vi "Rinocloud_lab_simulator.vi"() -> ()   [LabVIEW 2011, in "Rinocloud Library.lvlib"]
uses:
  Rinocloud Library.lvlib
  <vilib>/Utility/miscctls.llb/LVDateTimeRec.ctl
  Rinocloud_global_variable.vi
panel:
  in  "Active item:":string
  in  "image":bool
  out "Data saved":bool
  in  "extra information field 2":T1={"Attribute"="Sample ID", "Value"="A2008", "Data type"=enum."String"}
  in  "extra information field 3":T1={"Attribute"="Units", "Value"="nm,cps", "Data type"=enum."1D array of strings"}
  in  "notes":string="Rino client testing"
  in  "tags":string="1D data, testing"
  in  "name":string="Measurements"
  in  "extra information field":T1={"Attribute"="Labels", "Value"="Timestamp,Amplitude", "Data type"=enum."1D array of strings"}
  out "data JSON string":string="[[], []]"
  in  "Run":bool
  in  "Save":bool
  in  "X axis type:":u16(ring) items=["numerical"]
  out "headers":string
  out "body":string
  out "XY Graph":cluster{"x axis":dbl[], "x axis":dbl[]}[](graph)
  out "output array":cluster{"x axis":dbl[], "2D data":dbl[]}[](array[cluster])
  out "x axis":dbl[](array[numeric])
  out "1D data":dbl[](array[numeric])
  out "Array":dbl[](array[numeric])
  out "z axis":dbl[](array[numeric])
  out "2D data":dbl[][](array[numeric])
  out "x timestamps":string[](array[string])
  out "x native timestamp":timestamp[](array[timestamp])
  in  "stop":bool
  in  "Data type:":u16(ring) items=["1D array", "2D array"]
  # ":"
  # "{\"Attribute\" : \"Value\"}"
  # ":"
  # "{\"Attribute\" : \"Value\"}"
  # ":"
  # "{\"Attribute\" : \"Value\"}"
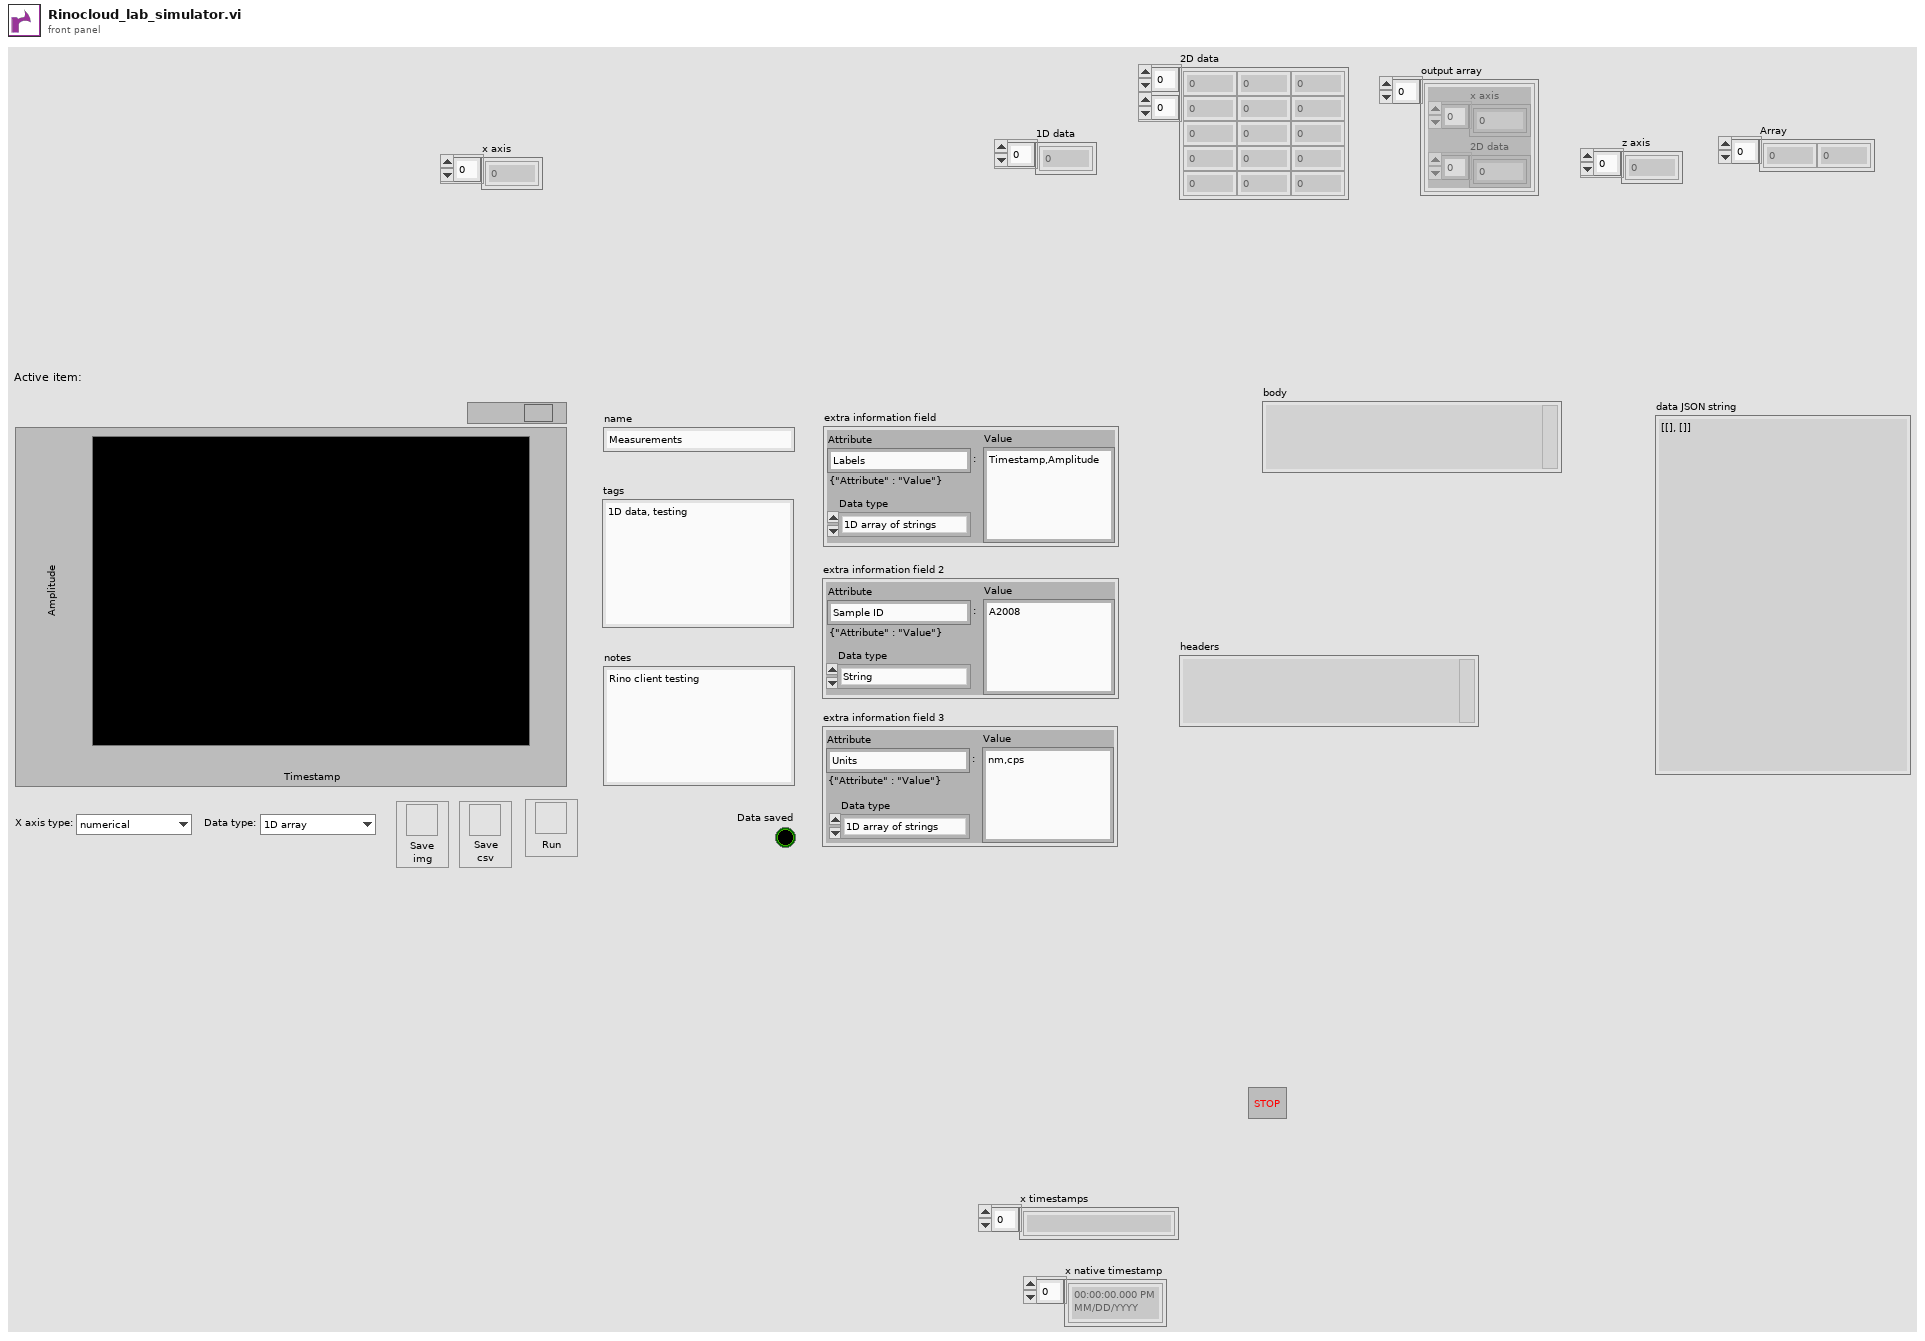
[diagram p1: front panel]
types:
  T1 = cluster{"Attribute":string, "Value":string, "Data type":enum16{"Numeric", "String", "1D array of strings", "1D array of doubles", "Data JSON string", "<null>"}}
  T2 = typedef "LVDateTimeRec.ctl" = cluster{"fractional second":dbl, "second":i32, "minute":i32, "hour":i32, "day of month":i32, "month":i32, "year":i32, "day of week":i32, "day of year":i32, "DST":i32}
  T3 = cluster{"Attribute":string, "Value":string, "Data type":enum16{"Numeric", "String", "1D array of strings", "1D array of doubles", "Data JSON string", "<null>"}}[]
  T4 = cluster{"headers":string, "body":string, "ID":string, "Saved":bool}
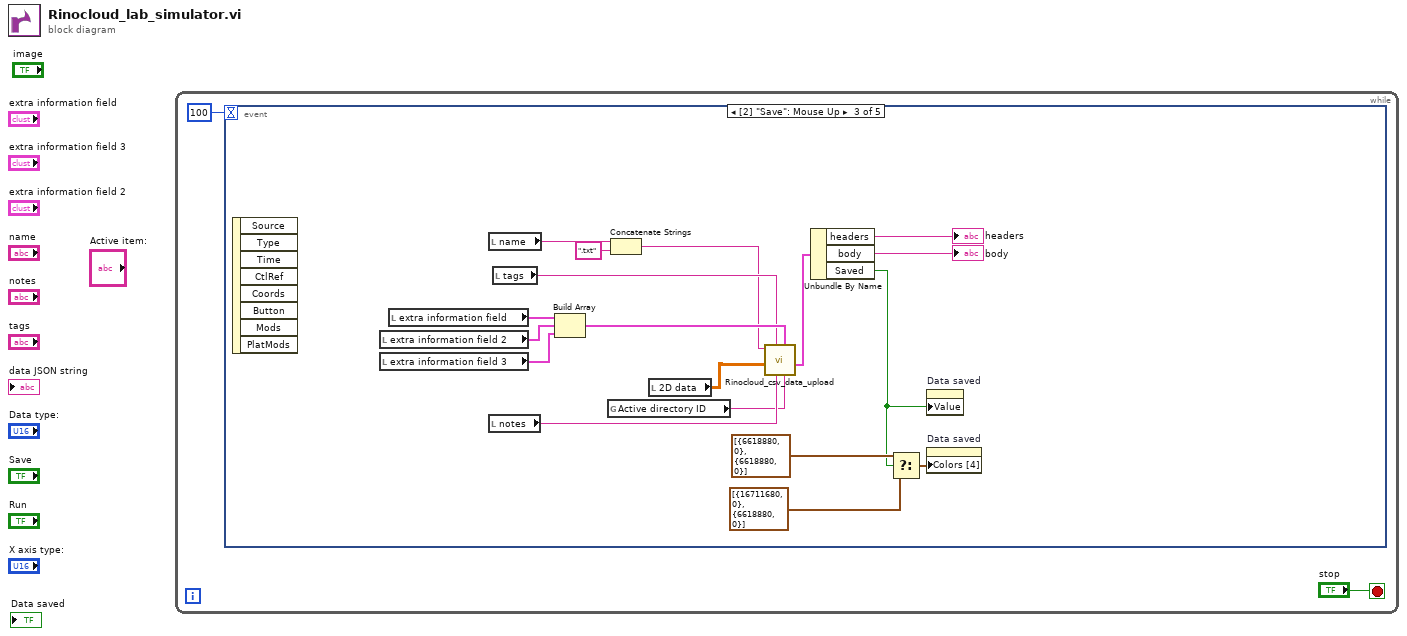
[diagram p0: block diagram]
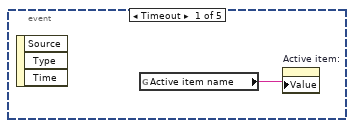
[diagram p2: hidden frame]
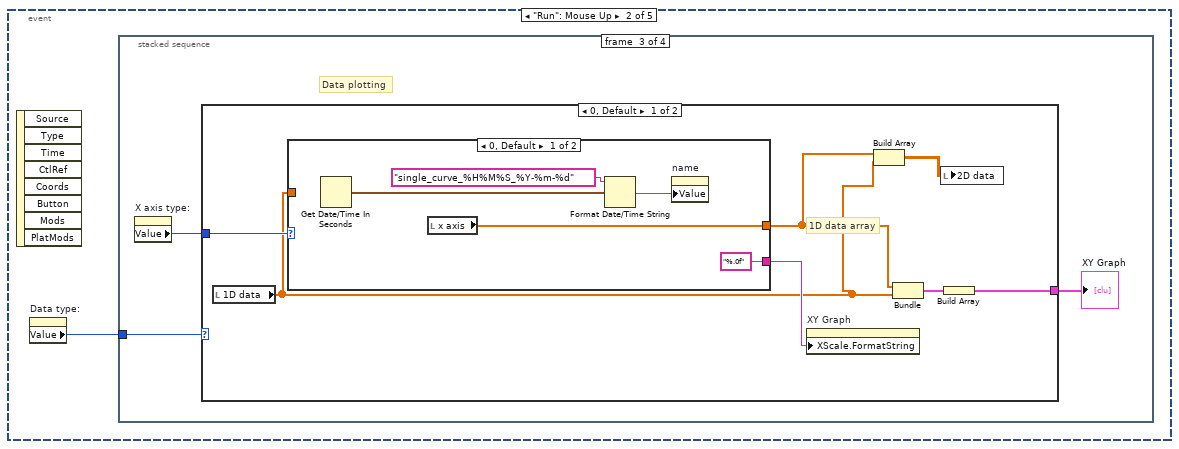
[diagram p3: hidden frame]
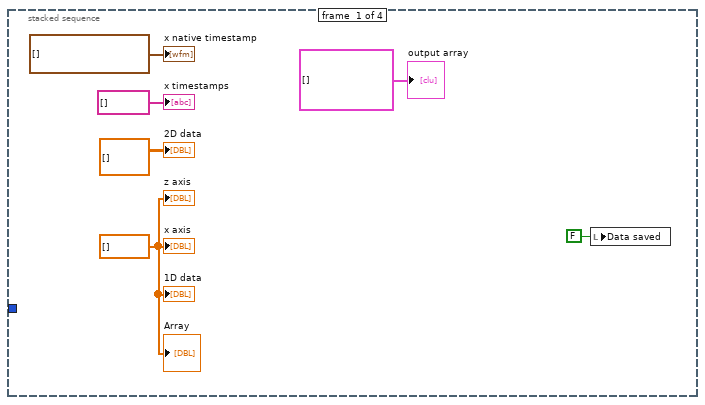
[diagram p4: hidden frame]
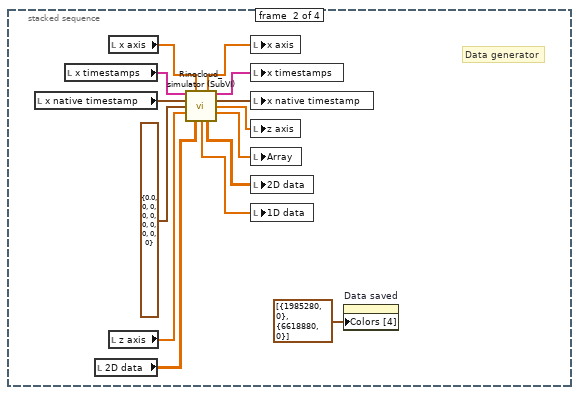
[diagram p5: hidden frame]
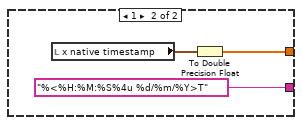
[diagram p6: hidden frame]
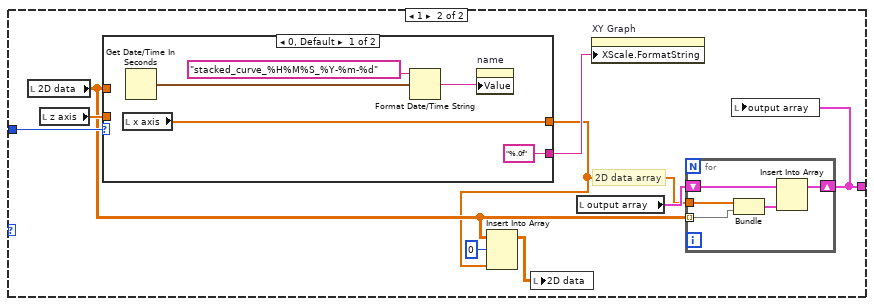
[diagram p7: hidden frame]
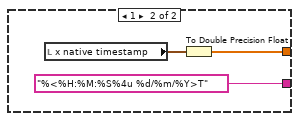
[diagram p8: hidden frame]
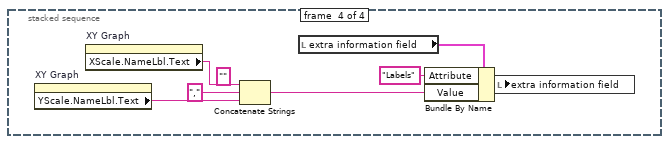
[diagram p9: hidden frame]
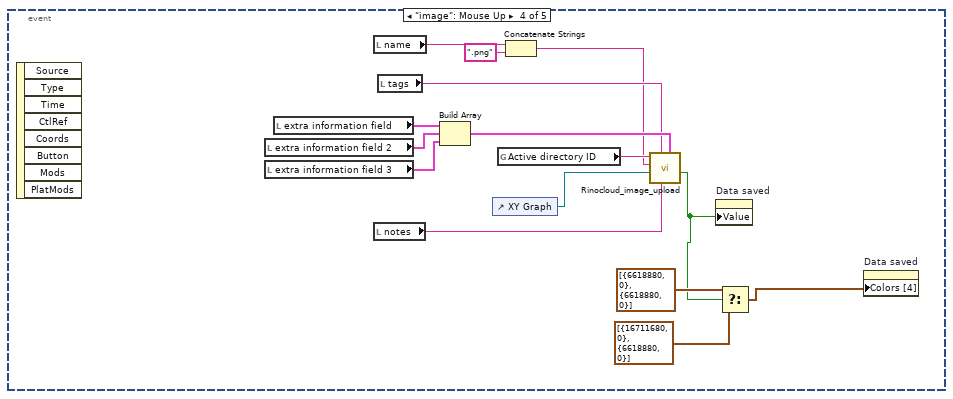
[diagram p10: hidden frame]
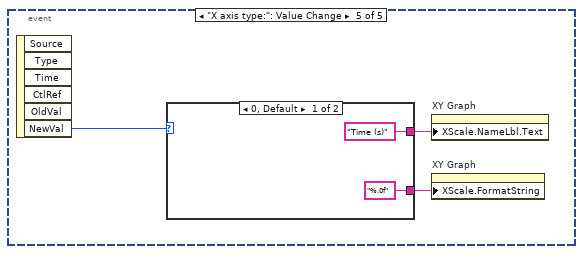
[diagram p11: hidden frame]
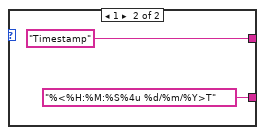
[diagram p12: hidden frame]
diagram:
  n1 = while {
    stop <- "stop" stop-if-true
    n2 = event shown="[2] \"Save\": Mouse Up" {
      selector: _ -> [_ _ _ _ _]
      dyn-events: _ -> [_ _ _ _ _]
      timeout: 100 -> [_ _ _ _ _]
      event Timeout {
        n3 = event-data() -> ()  [unwired: 1 in, 3 out]
        n4 = global read "Rinocloud_global_variable.vi" "Active item name"() -> (w3:string)
        n5 = property on="Active item:" class="Str"("Value"=w3) -> ()  [unwired: 2 in, 2 out]
      }
      event "Run": Mouse Up {
        n6 = event-data() -> ()  [unwired: 1 in, 8 out]
        n7 = property on="Data type:" class="Ring (strict)"() -> ("Value"=w4:u16)  [unwired: 2 in, 2 out]
        n8 = stacked-sequence {
          tunnel: w4 -> [_ _ w27 _]
          frame #0 {
            w9 = dbl[] []
            n9 = local write "Data saved"(FALSE ("Data saved")) -> ()
            "output array" <- cluster{"x axis":dbl[], "2D data":dbl[]}[] [] ("output array")
            "x axis" <- w9
            "1D data" <- w9
            "Array" <- w9
            "z axis" <- w9
            "2D data" <- dbl[][] []
            "x timestamps" <- string[] [] ("x timestamps")
            "x native timestamp" <- timestamp[] [] ("x native timestamp")
          }
          frame #1 {
            # "Data generator"
            n10 = local read "x native timestamp"() -> (w14:timestamp[])
            n11 = local read "x timestamps"() -> (w16:string[])
            n12 = local read "2D data"() -> (w23:dbl[][])
            n13 = local read "x axis"() -> (w24:dbl[])
            n14 = local read "z axis"() -> (w18:dbl[])
            n15 = call "Rinocloud_simulator (SubVI).vi"("x timestamps in"=w16, "x axis in"=w24, "x native timestamp in"=w14, "date time rec"=T2 {"fractional second"=0.0, "second"=0, "minute"=0, "hour"=0, "day of month"=0, "month"=0, "year"=0, "day of week"=0, "day of year"=0, "DST"=0}, "z axis in"=w18, "2D data in"=w23) -> ("x axis out"=w19:dbl[], "x timestamps out"=w15:string[], "x native timestamp out"=w13:timestamp[], "z axis out"=w17:dbl[], "Array 2"=w21:dbl[], "Array"=w20:dbl[], "2D data out"=w22:dbl[][])  [unwired: 3 in]
            n16 = local write "x axis"(w19) -> ()
            n17 = local write "x timestamps"(w15) -> ()
            n18 = local write "x native timestamp"(w13) -> ()
            n19 = local write "z axis"(w17) -> ()
            n20 = local write "Array"(w21) -> ()
            n21 = local write "2D data"(w22) -> ()
            n22 = local write "1D data"(w20) -> ()
            n23 = property on="Data saved" class="Bool (strict)"("Colors [4]"=cluster{u32, u32}[] [{1985280, 0}, {6618880, 0}]) -> ()  [unwired: 2 in, 2 out]
          }
          frame #2 {
            # "Data plotting"
            n24 = property on="X axis type:" class="Ring (strict)"() -> ("Value"=w25:u16)  [unwired: 2 in, 2 out]
            n25 = case shown="0, Default" w27 {
              tunnel: [w33 w50] -> w26
              tunnel: w25 -> [w32 w48]
              frame 0, Default {
                # "1D data array"
                n26 = local read "1D data"() -> (w29:dbl[])
                n27 = case shown="0, Default" w32 {
                  tunnel: [w38 w40] -> w30
                  tunnel: ["%.0f" ("X Scale.Format String") "%<%H:%M:%S%4u %d/%m/%Y>T" ("X Scale.Format String")] -> w31
                  tunnel: w29 -> [_ _]
                  frame 0, Default {
                    n28 = Get Date/Time In Seconds() -> (seconds since 1Jan1904=w37:timestamp)
                    n29 = local read "x axis"() -> (w38:dbl[])
                    n30 = Format Date/Time String(time format string (%c)="single_curve_%H%M%S_%Y-%m-%d", seconds (now)=w37) -> (date/time string=w36:string)  [unwired: 1 in]
                    n31 = property on="name" class="Str"("Value"=w36) -> ()  [unwired: 2 in, 2 out]
                  }
                  frame 1 {
                    n32 = local read "x native timestamp"() -> (w41:timestamp[])
                    n33 = To Double Precision Float(number=w41) -> (double precision float=w40:dbl[])
                  }
                }
                n34 = property on="XY Graph" class="XYGraph (strict)"("XScale.FormatString"=w31) -> ()  [unwired: 2 in, 2 out]
                n35 = Build Array(w30, w29) -> (w28:dbl[][])
                n36 = Bundle("x axis"=w30, "1D data"=w29) -> (w34:cluster{"x axis":dbl[], "1D data":dbl[]})  [unwired: 1 in]
                n37 = local write "2D data"(w28) -> ()
                n38 = Build Array(w34) -> (w33:cluster{"x axis":dbl[], "1D data":dbl[]}[])
              }
              frame 1 {
                # "2D data array"
                n39 = local read "2D data"() -> (w44:dbl[][])
                n40 = local read "z axis"() -> (w47:dbl[])
                n41 = case shown="0, Default" w48 {
                  tunnel: [w55 w57] -> w43
                  tunnel: ["%.0f" ("X Scale.Format String") "%<%H:%M:%S%4u %d/%m/%Y>T" ("X Scale.Format String")] -> w49
                  tunnel: w47 -> [_ _]
                  tunnel: w44 -> [_ _]
                  frame 0, Default {
                    n42 = local read "x axis"() -> (w55:dbl[])
                    n43 = Get Date/Time In Seconds() -> (seconds since 1Jan1904=w53:timestamp)
                    n44 = Format Date/Time String(time format string (%c)="stacked_curve_%H%M%S_%Y-%m-%d", seconds (now)=w53) -> (date/time string=w52:string)  [unwired: 1 in]
                    n45 = property on="name" class="Str"("Value"=w52) -> ()  [unwired: 2 in, 2 out]
                  }
                  frame 1 {
                    n46 = local read "x native timestamp"() -> (w58:timestamp[])
                    n47 = To Double Precision Float(number=w58) -> (double precision float=w57:dbl[])
                  }
                }
                n48 = Insert Into Array(array=w44, index (row)=0, new element=w43) -> (w46:dbl[][])  [unwired: 1 in]
                n49 = local write "2D data"(w46) -> ()
                n50 = local read "output array"() -> (w51:cluster{"x axis":dbl[], "2D data":dbl[]}[])
                n51 = property on="XY Graph" class="XYGraph (strict)"("XScale.FormatString"=w49) -> ()  [unwired: 2 in, 2 out]
                n52 = for {
                  tunnel: w44 -> [w63] mode=indexing
                  tunnel: w43 -> [w64]
                  shift-right: [w61] -> w50
                  shift-left: w51 -> [w60]
                  n53 = Bundle("x axis"=w64, "2D data"=w63) -> (w62:cluster{"x axis":dbl[], "2D data":dbl[]})  [unwired: 1 in]
                  n54 = Insert Into Array(array=w60, new element=w62) -> (w61:cluster{"x axis":dbl[], "2D data":dbl[]}[])  [unwired: 1 in]
                }
                n55 = local write "output array"(w50) -> ()
              }
            }
            "XY Graph" <- w26
          }
          frame #3 {
            (unwired) "" ("string")
            n56 = property on="XY Graph" class="XYGraph (strict)"() -> ("YScale.NameLbl.Text"=w69:string)  [unwired: 2 in, 2 out]
            n57 = property on="XY Graph" class="XYGraph (strict)"() -> ("XScale.NameLbl.Text"=w71:string)  [unwired: 2 in, 2 out]
            n58 = Concatenate Strings(w71, "," ("string"), w69) -> (w67:string)
            n59 = local read "extra information field"() -> (w68:T1)
            n60 = Bundle By Name(cluster=w68, "Attribute"="Labels" ("Key 1"), "Value"=w67) -> (w65:T1)
            n61 = local write "extra information field"(w65) -> ()
          }
        }
      }
      event "Save": Mouse Up {
        n62 = event-data() -> ()  [unwired: 1 in, 8 out]
        n63 = local read "extra information field 2"() -> (w88:T1)
        n64 = local read "extra information field 3"() -> (w87:T1)
        n65 = local read "extra information field"() -> (w89:T1)
        n66 = local read "name"() -> (w84:string)
        n67 = local read "notes"() -> (w85:string)
        n68 = local read "tags"() -> (w78:string)
        n69 = Build Array(w89, w88, w87) -> (w86:T3)
        n70 = global read "Rinocloud_global_variable.vi" "Active directory ID"() -> (w77:string)
        n71 = Concatenate Strings(w84, ".txt" ("string")) -> (w76:string)
        n72 = local read "2D data"() -> (w82:dbl[][])
        n73 = call "Rinocloud_csv_data_upload.vi"("Parent ID"=w77, "Extra metadata array"=w86, "Notes"=w85, "Tags"=w78, "2D numerical data"=w82, "Name"=w76) -> ("Status"=w75:T4)  [unwired: 4 in, 1 out]
        n74 = Unbundle By Name(w75) -> ("headers"=→"headers":string, "body"=→"body":string, "Saved"=w74:bool)
        n75 = Select(t=cluster{u32, u32}[] [{6618880, 0}, {6618880, 0}] ("Colors [4]"), s=w74, f=cluster{u32, u32}[] [{16711680, 0}, {6618880, 0}] ("Colors [4]")) -> (s? t:f=w79:cluster{u32, u32}[])
        n76 = property on="Data saved" class="Bool (strict)"("Value"=w74) -> ()  [unwired: 2 in, 2 out]
        n77 = property on="Data saved" class="Bool (strict)"("Colors [4]"=w79) -> ()  [unwired: 2 in, 2 out]
      }
      event "image": Mouse Up {
        n78 = event-data() -> ()  [unwired: 1 in, 8 out]
        n79 = local read "extra information field 2"() -> (w103:T1)
        n80 = local read "extra information field 3"() -> (w102:T1)
        n81 = local read "extra information field"() -> (w104:T1)
        n82 = local read "name"() -> (w97:string)
        n83 = local read "notes"() -> (w98:string)
        n84 = local read "tags"() -> (w99:string)
        n85 = Build Array(w104, w103, w102) -> (w101:T3)
        n86 = control-ref of="XY Graph"() -> (w90:refnum<vi>)
        n87 = global read "Rinocloud_global_variable.vi" "Active directory ID"() -> (w100:string)
        n88 = Concatenate Strings(w97, ".png" ("string")) -> (w95:string)
        n89 = call "Rinocloud_image_upload.vi"("Extra metadata array"=w101, "Notes"=w98, "Tags"=w99, "Wavefrom Refnum"=w90, "Name"=w95, "Parent ID"=w100) -> ("Saved"=w91:bool)  [unwired: 2 in, 3 out]
        n90 = property on="Data saved" class="Bool (strict)"("Value"=w91) -> ()  [unwired: 2 in, 2 out]
        n91 = Select(t=cluster{u32, u32}[] [{6618880, 0}, {6618880, 0}] ("Colors [4]"), s=w91, f=cluster{u32, u32}[] [{16711680, 0}, {6618880, 0}] ("Colors [4]")) -> (s? t:f=w92:cluster{u32, u32}[])
        n92 = property on="Data saved" class="Bool (strict)"("Colors [4]"=w92) -> ()  [unwired: 2 in, 2 out]
      }
      event "X axis type:": Value Change {
        n93 = event-data() -> ("NewVal"=w107:u16)  [unwired: 1 in, 5 out]
        n94 = case shown="0, Default" w107 {
          tunnel: ["Time (s)" ("X Scale.Unit Label.Text") "Timestamp" ("X Scale.Unit Label.Text")] -> w106
          tunnel: ["%.0f" ("X Scale.Format String") "%<%H:%M:%S%4u %d/%m/%Y>T" ("X Scale.Format String")] -> w105
          frame 0, Default {
          }
          frame 1 {
          }
        }
        n95 = property on="XY Graph" class="XYGraph (strict)"("XScale.NameLbl.Text"=w106) -> ()  [unwired: 2 in, 2 out]
        n96 = property on="XY Graph" class="XYGraph (strict)"("XScale.FormatString"=w105) -> ()  [unwired: 2 in, 2 out]
      }
    }
  }
